vi "Usage.vi"() -> ()   [LabVIEW 2017]
uses:
  Message/Abstract Message/Abstract Message.lvclass
  Message Queue/Message Queue/Message Queue.lvclass
  <vilib>/Platform/TimedLoop/XDataNode/timing_clust.ctl
  <vilib>/Platform/TimedLoop/XDataNode/nitl_modes.ctl
  <vilib>/Platform/TimedLoop/XDataNode/wakeup.ctl
  Tests/Test Message/Test Message.lvclass
  C:/github/niveristand-custom-device-message-library/Source/Message/Abstract Message/Abstract Message.lvclass
  <vilib>/platform/TimedLoop/XDataNode/XDataNode.xnode
  <vilib>/Platform/TimedLoop/XDataNode/XDNodeRunTimeDep.lvlib
panel:
  in  "stop":bool
  out "Message out 2":refnum<class "Abstract Message.lvclass">
  out "Message out":refnum<class "Abstract Message.lvclass">
  out "maximum number of messages 2":i32
  out "current number of messages 2":i32
  out "error out 3":errorcluster
  out "error out 2":errorcluster
  out "current number of messages":i32
  out "maximum number of messages":i32
  out "error out":errorcluster
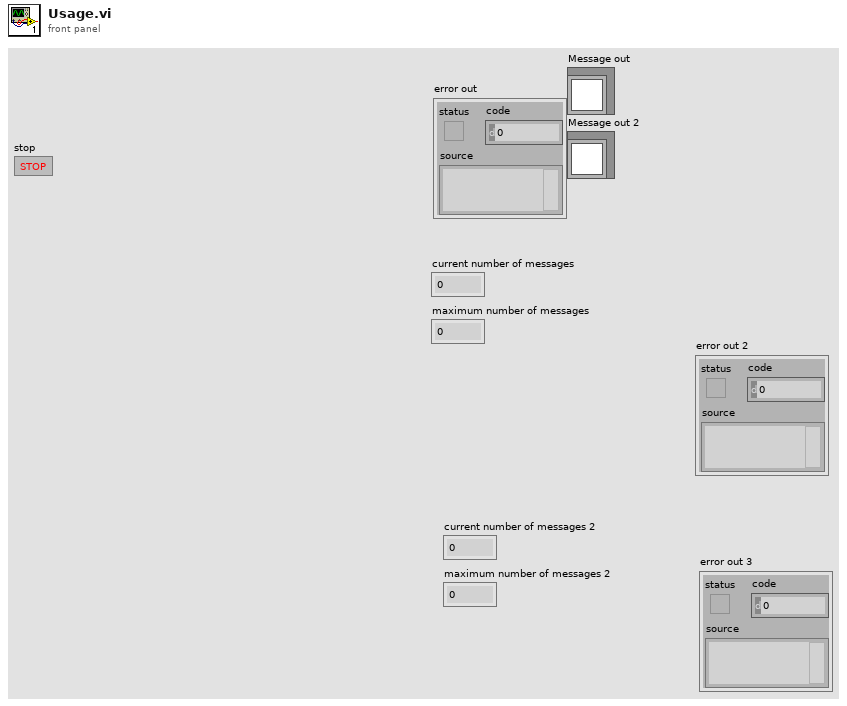
[diagram p1: front panel]
types:
  T1 = typedef "XDNodeRunTimeDep.lvlib/timing_clust.ctl" = cluster{"Expected End [f-1]":u64, "Actual End [f-1]":u64, "Finished Late? [f-1]":bool, "Expected End [i-1]":u64, "Actual End [i-1]":u64, "Finished Late? [i-1]":bool, "Expected Start [i]":u64, "Actual Start [i]":u64, "Expected Start [f]":u64, "Actual Start [f]":u64, "Source Name":string, "Structure Name":string, "Period":i64, "Deadline":i64, "Offset":i64, "Start":i64, "Priority":i32, "Timeout":i32, "Mode":T2, "Wakeup Reason":T3, "Error":errorcluster, "Source Type":string, "Secondary Source Type":string, "Global End Time":u64, "Global Start Time":u64, "Frame Duration":u64, "Iteration Duration":u64, "Assigned CPU":i32, "I/O Scan Engine Mode":u32}
  T2 = typedef "XDNodeRunTimeDep.lvlib/nitl_modes.ctl" = enum32{"No Change", "Process missed periods, maintain original phase", "Discard missed periods, maintain original phase", "Process missed periods, ignore original phase", "Discard missed periods, ignore original phase"}
  T3 = typedef "XDNodeRunTimeDep.lvlib/wakeup.ctl" = enum32{"Normal", "Aborted", "Asynchronous wakeup", "Timing source error", "Timed loop error", "Timeout"}
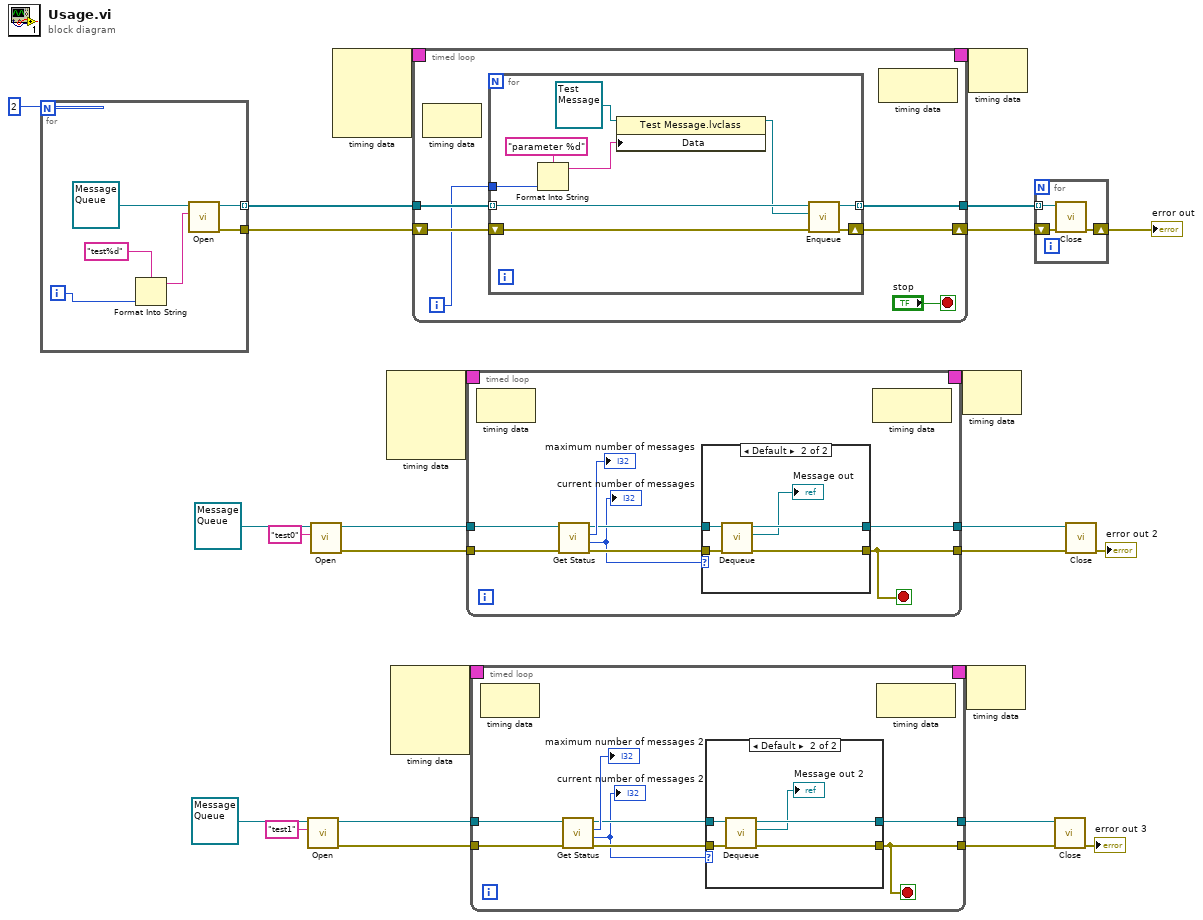
[diagram p0: block diagram]
diagram:
  n1 = for {
    N: 2 -> [_]
    tunnel: [w31] -> w7 mode=indexing
    tunnel: [w30] -> w24
    i -> [w29]
    n2 = Format Into String(format string="test%d", w29) -> (resulting string=w28:string)  [unwired: 2 in, 1 out]
    n3 = call-dynamic "Open.vi"("name (unnamed)"=w28, "Message Queue in"=refnum<class "Message Queue.lvclass"> refnum ("Message Library.lvlib:FIFO.lvclass")) -> ("error out"=w30:errorcluster, "Message Queue out"=w31:refnum<class "Message Queue.lvclass">)  [unwired: 8 in]
  }
  n4 = call-dynamic "Open.vi"("name (unnamed)"="test1", "Message Queue in"=refnum<class "Message Queue.lvclass"> refnum ("Message Library.lvlib:FIFO.lvclass")) -> ("error out"=w3:errorcluster, "Message Queue out"=w4:refnum<class "Message Queue.lvclass">)  [unwired: 8 in]
  n5 = call-dynamic "Open.vi"("name (unnamed)"="test0", "Message Queue in"=refnum<class "Message Queue.lvclass"> refnum ("Message Library.lvlib:FIFO.lvclass")) -> ("error out"=w16:errorcluster, "Message Queue out"=w17:refnum<class "Message Queue.lvclass">)  [unwired: 8 in]
  n6 = node-c288() -> (w26:T1)  [unwired: 4 in]
  n7 = node-c288() -> (w20:T1)  [unwired: 4 in]
  n8 = node-c288() -> (w6:T1)  [unwired: 4 in]
  n9 = timed-loop {
    timing: w26 -> [_]
    timing-out: [_] -> w25
    tunnel: w7 -> [w35]
    shift-right: [w37] -> w22
    shift-left: w24 -> [w38]
    tunnel: [w36] -> w23
    i -> [w34]
    stop <- "stop" stop-if-true
    n10 = node-c288() -> ()  [unwired: 1 in, 1 out]
    n11 = for {
      tunnel: [w47] -> w36 mode=indexing
      tunnel: w35 -> [w46] mode=indexing
      shift-right: [w48] -> w37
      shift-left: w38 -> [w49]
      tunnel: w34 -> [w44]
      n12 = Format Into String(format string="parameter %d", w44) -> (resulting string=w43:string)  [unwired: 2 in, 1 out]
      n13 = property class="Test Message.lvclass"(reference=refnum<class "Test Message.lvclass"> refnum ("Message Queue Library.lvlib:Test Message.lvclass"), "Data"=w43) -> (reference out=w41:refnum<class "Test Message.lvclass">)  [unwired: 1 in, 1 out]
      n14 = call-dynamic "Enqueue.vi"("error in (no error)"=w49, "Message in"=w41, "Message Queue in"=w46) -> ("error out"=w48:errorcluster, "Message Queue out"=w47:refnum<class "Message Queue.lvclass">)  [unwired: 7 in]
    }
    n15 = node-c288() -> ()  [unwired: 1 in, 1 out]
  }
  n16 = timed-loop {
    timing: w20 -> [_]
    timing-out: [_] -> w19
    tunnel: w17 -> [w57]
    tunnel: w16 -> [w56]
    tunnel: [w53] -> w15
    tunnel: [w51] -> w14
    stop <- w51 stop-if-true
    n17 = node-c288() -> ()  [unwired: 1 in, 1 out]
    n18 = call-dynamic "Get Status.vi"("error in (no error)"=w56, "Message Queue in"=w57) -> ("error out"=w52:errorcluster, "current number of messages"=w50:i32, "maximum number of messages"=→"maximum number of messages":i32, "Message Queue out"=w54:refnum<class "Message Queue.lvclass">)  [unwired: 6 in]
    "current number of messages" <- w50
    n19 = case shown="Default" w50 {
      tunnel: w54 -> [w59 w64]
      tunnel: [w59 w63] -> w53
      tunnel: w52 -> [w58 w62]
      tunnel: [w58 w61] -> w51
      frame 0 {
      }
      frame Default {
        n20 = call-dynamic "Dequeue.vi"("error in (no error)"=w62, "Message Queue in"=w64) -> ("error out"=w61:errorcluster, "Message out"=→"Message out":refnum<class "Abstract Message.lvclass">, "Message Queue out"=w63:refnum<class "Message Queue.lvclass">)  [unwired: 7 in]
      }
    }
    n21 = node-c288() -> ()  [unwired: 1 in, 1 out]
  }
  n22 = timed-loop {
    timing: w6 -> [_]
    timing-out: [_] -> w5
    tunnel: w4 -> [w74]
    tunnel: w3 -> [w73]
    tunnel: [w70] -> w2
    tunnel: [w68] -> w1
    stop <- w68 stop-if-true
    n23 = node-c288() -> ()  [unwired: 1 in, 1 out]
    n24 = call-dynamic "Get Status.vi"("error in (no error)"=w73, "Message Queue in"=w74) -> ("error out"=w69:errorcluster, "current number of messages"=w67:i32, "maximum number of messages"=→"maximum number of messages 2":i32, "Message Queue out"=w71:refnum<class "Message Queue.lvclass">)  [unwired: 6 in]
    "current number of messages 2" <- w67
    n25 = case shown="Default" w67 {
      tunnel: w71 -> [w76 w81]
      tunnel: [w76 w80] -> w70
      tunnel: w69 -> [w75 w79]
      tunnel: [w75 w78] -> w68
      frame 0 {
      }
      frame Default {
        n26 = call-dynamic "Dequeue.vi"("error in (no error)"=w79, "Message Queue in"=w81) -> ("error out"=w78:errorcluster, "Message out"=→"Message out 2":refnum<class "Abstract Message.lvclass">, "Message Queue out"=w80:refnum<class "Message Queue.lvclass">)  [unwired: 7 in]
      }
    }
    n27 = node-c288() -> ()  [unwired: 1 in, 1 out]
  }
  n28 = node-c288(w19) -> ()  [unwired: 1 out]
  n29 = node-c288(w5) -> ()  [unwired: 1 out]
  n30 = node-c288(w25) -> ()  [unwired: 1 out]
  n31 = for {
    tunnel: w23 -> [w86] mode=indexing
    shift-right: [w84] -> w21
    shift-left: w22 -> [w85]
    n32 = call-dynamic "Close.vi"("error in (no error)"=w85, "Message Queue in"=w86) -> ("error out"=w84:errorcluster)  [unwired: 8 in, 1 out]
  }
  "error out" <- w21
  n33 = call-dynamic "Close.vi"("error in (no error)"=w1, "Message Queue in"=w2) -> ("error out"=→"error out 3":errorcluster)  [unwired: 8 in, 1 out]
  n34 = call-dynamic "Close.vi"("error in (no error)"=w14, "Message Queue in"=w15) -> ("error out"=→"error out 2":errorcluster)  [unwired: 8 in, 1 out]
